vi "Read Logger.vi"(11 "Proccess in":refnum<class "Proccess.lvclass">) -> (2 "Logger":refnum<class "Logger.lvclass">)   [LabVIEW 2019, in "Proccess.lvclass"]
uses:
  Proccess.lvclass
  Logger_class/Logger.lvclass
  Proccess.lvclass/Proccess.ctl
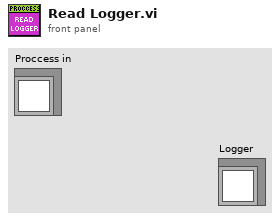
[diagram p1: front panel]
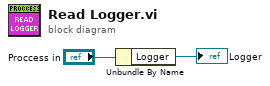
[diagram p0: block diagram]
diagram:
  n1 = Unbundle By Name("Proccess in") -> ("Logger"=→"Logger":refnum<class "Logger.lvclass">)
